vi "Write controls.vi"(5 "controls":variant, 9 "PythonConverter_GUI in":refnum<class "PythonConverter_GUI.lvclass">) -> (3 "PythonConverter_GUI out":refnum<class "PythonConverter_GUI.lvclass">)   [LabVIEW 2014, in "Raspberry Pi Compatible Compiler for LabVIEW.lvlib" / "PythonConverter_GUI.lvclass"]
uses:
  PythonConverter_GUI.lvclass
  PythonConverter_GUI.lvclass/PythonConverter_GUI.ctl
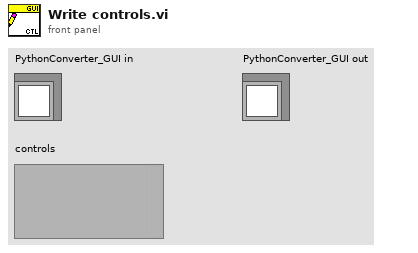
[diagram p1: front panel]
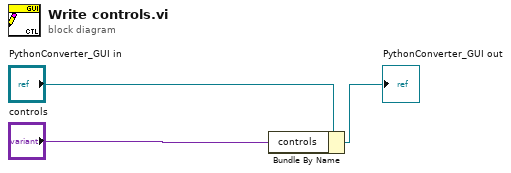
[diagram p0: block diagram]
diagram:
  n1 = Bundle By Name(cluster="PythonConverter_GUI in", "controls"="controls") -> (→"PythonConverter_GUI out":refnum<class "PythonConverter_GUI.lvclass">)
